vi "dvp Vi Set Trigger Input Type.vi"(10 "TriggerInputType":u32(ring) items=["TRIGGER_IN_OFF", "TRIGGER_NEG_EDGE", "TRIGGER_LOW_LEVEL", "TRIGGER_POS_EDGE", "TRIGGER_HIGH_LEVEL"], 11 "handle":u32) -> (3 "function return":u32(ring))   [LabVIEW 2018, in "LabViewDVPCamera.lvlib"]
doc: "LabviewDvp2Api dvpStatus dvpViSetTriggerInputType(dvpHandle handle, dvpTriggerInputType TriggerInputType);"
uses:
  LabViewDVPCamera.lvlib
  LabViewDVPCamera/LabViewDVPCamera.dll
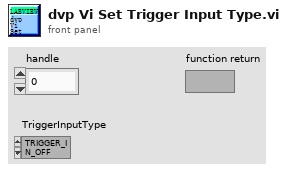
[diagram p1: front panel]
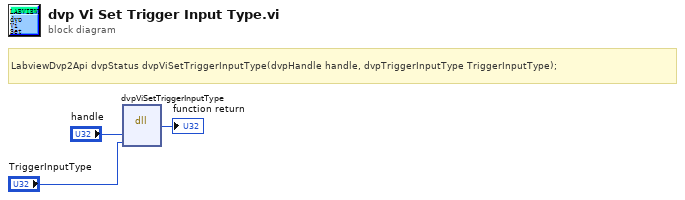
[diagram p0: block diagram]
diagram:
  # "LabviewDvp2Api dvpStatus dvpViSetTriggerInputType(dvpHandle handle, dvpTriggerInputType TriggerInputType);"
  n1 = dll-call lib="C:/Program Files (x86)/DVP2 Labview cn 64/Sample/LabViewDVPCamera/LabViewDVPCamera.*" fn="dvpViSetTriggerInputType"("handle"="handle", "TriggerInputType"="TriggerInputType") -> (→"function return":u32)  [unwired: 5 in, 2 out]
